vi "Sans titre 8.vi"() -> ()   [LabVIEW 2017]
uses:
  <vilib>/Field R&D Services/LIBSSH2 for LabVIEW/Toolkit/SSH/SSH.lvclass
  <vilib>/Field R&D Services/LIBSSH2 for LabVIEW/Toolkit/Session/Session.lvclass
  <vilib>/Field R&D Services/LIBSSH2 for LabVIEW/Toolkit/Session/Support/Create from SSH.vi
  <vilib>/Field R&D Services/LIBSSH2 for LabVIEW/Toolkit/Channel/Channel.lvclass
  <vilib>/Field R&D Services/LIBSSH2 for LabVIEW/Toolkit/Channel/Support/Create from Session.vi
  <vilib>/Field R&D Services/LIBSSH2 for LabVIEW/Toolkit/Channel/Support/Destroy to Session.vi
  <vilib>/Field R&D Services/LIBSSH2 for LabVIEW/Toolkit/Session/Support/Destroy to SSH.vi
  <vilib>/Field R&D Services/LIBSSH2 for LabVIEW/Toolkit/Session/Support/Public Key Memory Authentication.vi
  <vilib>/Field R&D Services/LIBSSH2 for LabVIEW/Toolkit/Field_RnD_Services_LIBSSH2_Toolkit.lvlib
panel:
  out "chaîne":string
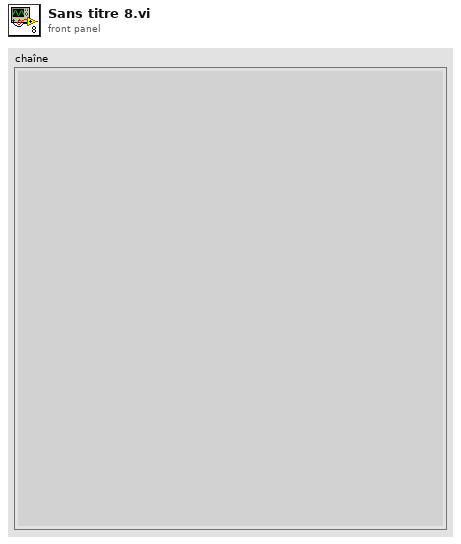
[diagram p1: front panel]
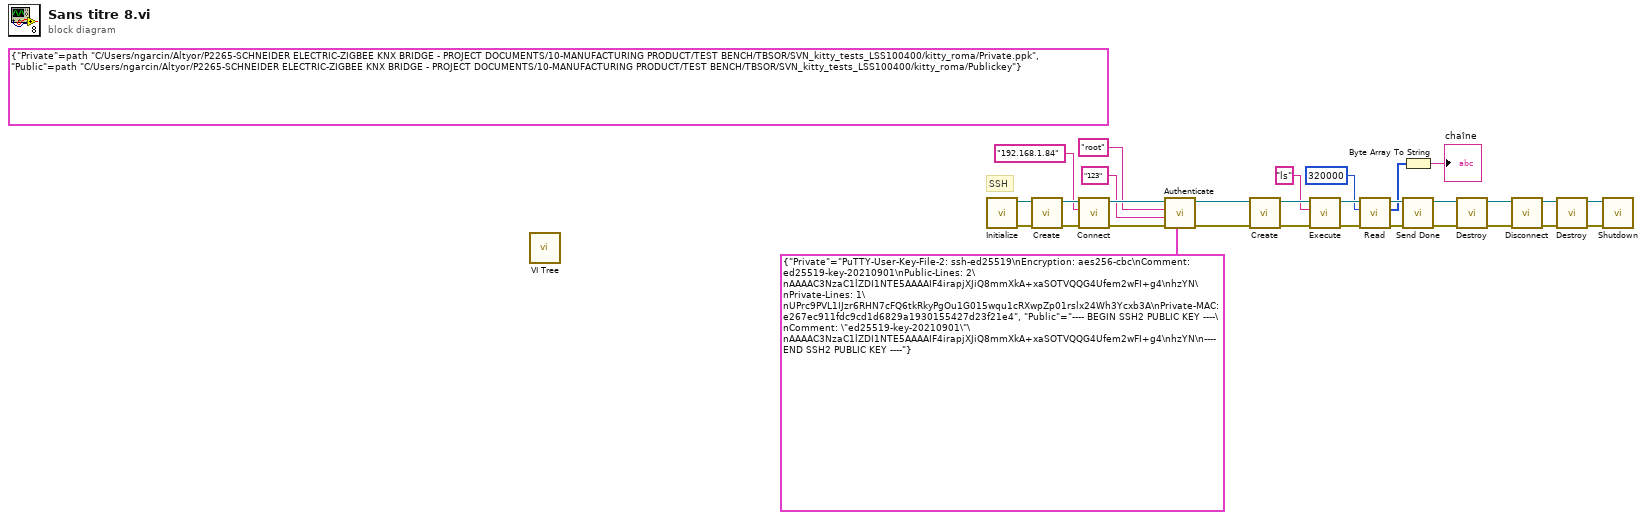
[diagram p0: block diagram]
diagram:
  (unwired) cluster{"Private":path, "Public":path} {"Private"=path "C:/Users/ngarcin/Altyor/P2265-SCHNEIDER ELECTRIC-ZIGBEE KNX BRIDGE - PROJECT DOCUMENTS/10-MANUFACTURING PRODUCT/TEST BENCH/TBSOR/SVN_kitty_tests_LSS100400/kitty_roma/Private.ppk", "Public"=path "C:/Users/ngarcin/Altyor/P2265-SCHNEIDER ELECTRIC-ZIGBEE KNX BRIDGE - PROJECT DOCUMENTS/10-MANUFACTURING PRODUCT/TEST BENCH/TBSOR/SVN_kitty_tests_LSS100400/kitty_roma/Publickey"} ("Keys")
  # "SSH"
  n1 = call <vilib>:"VI Tree.vi"() -> ()  [unwired: 12 in]
  n2 = call <vilib>:"Initialize.vi"() -> ("Error Out"=w29:errorcluster, "SSH"=w30:refnum<class "SSH.lvclass">)  [unwired: 10 in]
  n3 = call-poly <vilib>:"Create.vi"("Error In"=w29, "SSH"=w30) -> ("Error Out"=w28:errorcluster, "Sesssion"=w27:refnum<class "Session.lvclass">)  [unwired: 8 in]
  n4 = call <vilib>:"Connect.vi"("Error In"=w28, "Address"="192.168.1.84", "Session In"=w27) -> ("Error Out"=w25:errorcluster, "Sesssion Out"=w26:refnum<class "Session.lvclass">)  [unwired: 7 in]
  n5 = call-poly <vilib>:"Authenticate.vi"("Keys"=cluster{"Private":string, "Public":string} {"Private"="PuTTY-User-Key-File-2: ssh-ed25519\nEncryption: aes256-cbc\nComment: ed25519-key-20210901\nPublic-Lines: 2\nAAAAC3NzaC1lZDI1NTE5AAAAIF4irapjXJiQ8mmXkA+xaSOTVQQG4Ufem2wFI+g4\nhzYN\nPrivate-Lines: 1\nUPrc9PVL1IJzr6RHN7cFQ6tkRkyPgOu1G015wqu1cRXwpZp01rslx24Wh3Ycxb3A\nPrivate-MAC: e267ec911fdc9cd1d6829a1930155427d23f21e4", "Public"="---- BEGIN SSH2 PUBLIC KEY ----\nComment: \"ed25519-key-20210901\"\nAAAAC3NzaC1lZDI1NTE5AAAAIF4irapjXJiQ8mmXkA+xaSOTVQQG4Ufem2wFI+g4\nhzYN\n---- END SSH2 PUBLIC KEY ----"}, "Error In"=w25, "Passphrase"="123", "Username"="root", "Session In"=w26) -> ("Error Out"=w23:errorcluster, "Sesssion Out"=w24:refnum<class "Session.lvclass">)  [unwired: 5 in]
  n6 = call-poly <vilib>:"Create.vi"("Error In"=w23, "Session"=w24) -> ("Error Out"=w21:errorcluster, "Channel"=w22:refnum<class "Channel.lvclass">)  [unwired: 8 in]
  n7 = call <vilib>:"Execute.vi"("Error In"=w21, "Command"="ls", "Channel In"=w22) -> ("Error Out"=w20:errorcluster, "Channel Out"=w19:refnum<class "Channel.lvclass">)  [unwired: 7 in]
  n8 = call <vilib>:"Read.vi"("Error In"=w20, "Max Data Length"=u64 320000, "Channel In"=w19) -> ("Error Out"=w17:errorcluster, "Data"=w3:u8[], "Channel Out"=w18:refnum<class "Channel.lvclass">)  [unwired: 6 in]
  n9 = Byte Array To String(unsigned byte array=w3) -> (string=→"chaîne":string)
  n10 = call <vilib>:"Send Done.vi"("Error In"=w17, "Channel In"=w18) -> ("Error Out"=w9:errorcluster, "Channel Out"=w10:refnum<class "Channel.lvclass">)  [unwired: 8 in]
  n11 = call-poly <vilib>:"Destroy.vi"("Error In"=w9, "Channel"=w10) -> ("Error Out"=w15:errorcluster, "Session"=w16:refnum<class "Session.lvclass">)  [unwired: 8 in]
  n12 = call <vilib>:"Disconnect.vi"("Error In"=w15, "Session In"=w16) -> ("Error Out"=w12:errorcluster, "Sesssion Out"=w11:refnum<class "Session.lvclass">)  [unwired: 8 in]
  n13 = call-poly <vilib>:"Destroy.vi"("Error In"=w12, "Session"=w11) -> ("Error Out"=w13:errorcluster, "SSH"=w14:refnum<class "SSH.lvclass">)  [unwired: 8 in]
  n14 = call <vilib>:"Shutdown.vi"("Error In"=w13, "SSH"=w14) -> ()  [unwired: 9 in, 1 out]
